vi "api_GetAllParam.vi"(7 "group":string, 8 "error in (no error)":errorcluster, 11 "ConfigClass_DVR":refnum<data-value>) -> (0 "error out":errorcluster, 2 "params":string[](array[string]), 3 "ConfigClass_DVR_out":refnum<data-value>)   [LabVIEW 2019, in "ConfigClass.lvlib" / "ConfigClass.lvclass"]
uses:
  ConfigClass.lvclass
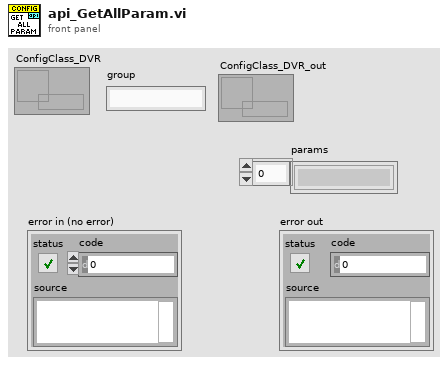
[diagram p1: front panel]
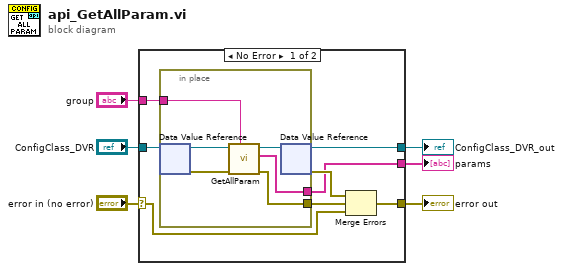
[diagram p0: block diagram]
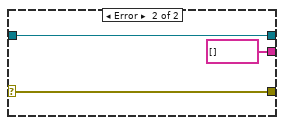
[diagram p2: hidden frame]
diagram:
  n1 = case shown="No Error" "error in (no error)" {
    selector: "error in (no error)" -> [w7 w23]
    tunnel: "ConfigClass_DVR" -> [w14 w22]
    tunnel: [w11 w23] -> w5
    tunnel: [w10 w22] -> w3
    tunnel: [w9 string[] [] ("params")] -> w2
    tunnel: "group" -> [w8 _]
    frame No Error {
      n2 = in-place {
        in-place-border: [w17] -> w12
        in-place-border: [w15] -> w9
        in-place-border: w8 -> [w20]
        n3 = in-place-dvr #1(w14) -> (w19:refnum<class "ConfigClass.lvclass">, w18:errorcluster)
        n4 = call-dynamic "GetAllParam.vi"("group"=w20, "error in (no error)"=w18, "ConfigClass_IN"=w19) -> ("error out"=w17:errorcluster, "params"=w15:string[], "ConfigClass_OUT"=w16:refnum<class "ConfigClass.lvclass">)  [unwired: 6 in]
        n5 = in-place-dvr #1(w16) -> (w10:refnum<data-value>, w13:errorcluster)
      }
      n6 = Merge Errors(w13, w12, w7) -> (w11:errorcluster)
    }
    frame Error {
    }
  }
  "ConfigClass_DVR_out" <- w3
  "error out" <- w5
  "params" <- w2
